vi "Handle Frame.vi"(8 "error in (no error)":errorcluster, 9 "Timeout ms":i32, 10 "Message Frame":T1, 11 "WebSocket Client in":refnum<class "WebSocket Client.lvclass">) -> (0 "error out":errorcluster, 1 "Remaining  Timeout":i32, 3 "WebSocket Client out":refnum<class "WebSocket Client.lvclass">, 4 "Complete":bool)   [LabVIEW 2020, in "HTTP Server.lvlib" / "WebSocket Client.lvclass"]
uses:
  WebSocket Client.lvclass
  WebSocket Client.lvclass/WebSocket Client.ctl
  OpCode.ctl
  Message Frame.ctl
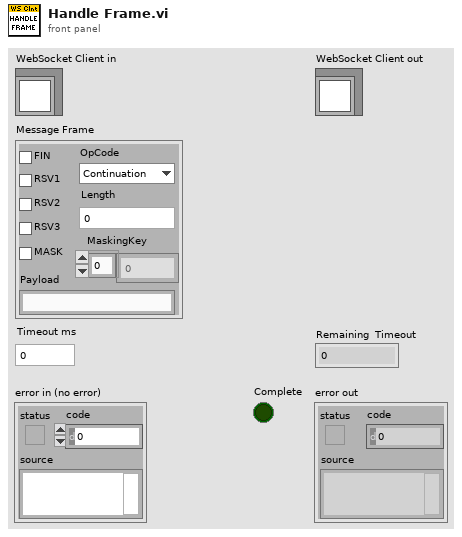
[diagram p1: front panel]
types:
  T1 = typedef "HTTP Server.lvlib/WebSocket Client.lvclass/Message Frame.ctl" = cluster{"FIN":bool, "RSV1":bool, "RSV2":bool, "RSV3":bool, "MASK":bool, "OpCode":T2, "Length":u64, "MaskingKey":u8[], "Payload":string}
  T2 = typedef "HTTP Server.lvlib/WebSocket Client.lvclass/OpCode.ctl" = enum8{"Continuation", "Text", "Binary", "Reserved3", "Reserved4", "Reserved5", "Reserved6", "Reserved7", "Close", "Ping", "Pong", "ReservedB", "ReservedC", "ReservedD", "ReservedE", "ReservedF"}
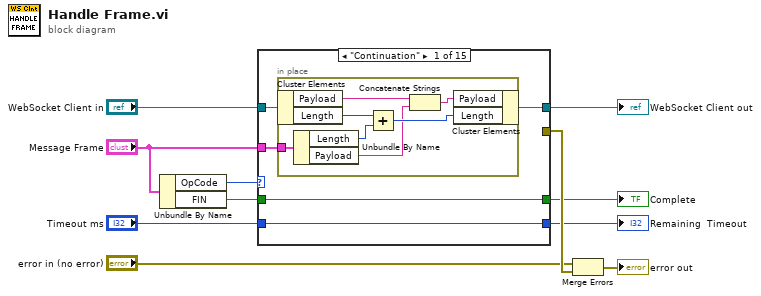
[diagram p0: block diagram]
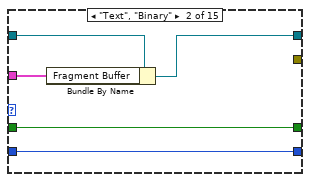
[diagram p2: hidden frame]
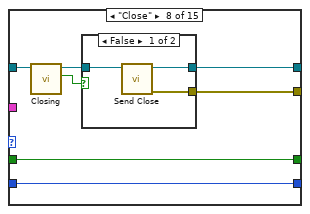
[diagram p8: hidden frame]
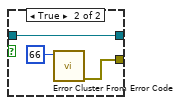
[diagram p9: hidden frame]
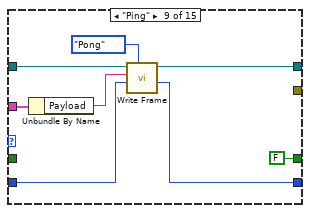
[diagram p10: hidden frame]
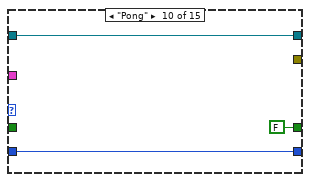
[diagram p11: hidden frame]
diagram:
  n1 = Unbundle By Name("Message Frame") -> ("OpCode"=w9:T2, "FIN"=w8:bool)
  n2 = case shown="\"Continuation\"" w9 {
    tunnel: w8 -> [w12 w27 w30 w33 w36 w39 w42 w49 _ _ w69 w72 w75 w78 w81]
    tunnel: "Timeout ms" -> [w16 w26 w29 w32 w35 w38 w41 w48 w60 w66 w68 w71 w74 w77 w80]
    tunnel: "WebSocket Client in" -> [w15 w28 w31 w34 w37 w40 w43 w50 w64 w67 w70 w73 w76 w79 w82]
    tunnel: [w13 w25 w31 w34 w37 w40 w43 w46 w63 w67 w70 w73 w76 w79 w82] -> w5
    tunnel: [w16 w26 w29 w32 w35 w38 w41 w48 w59 w66 w68 w71 w74 w77 w80] -> w4
    tunnel: "Message Frame" -> [w14 w24 _ _ _ _ _ _ w62 _ _ _ _ _ _]
    tunnel: [w12 w27 w30 w33 w36 w39 w42 w49 FALSE ("FIN") FALSE ("FIN") w69 w72 w75 w78 w81] -> w2
    tunnel: [_ _ _ _ _ _ _ w44 _ _ _ _ _ _ _] -> w11
    frame "Continuation" {
      n3 = in-place {
        in-place-border: w14 -> [w23]
        n4 = in-place-cluster #1(w15) -> ("Payload"=w19:string, "Length"=w22:u64)
        n5 = Unbundle By Name(w23) -> ("Length"=w21:u64, "Payload"=w18:string)
        n6 = Add(x=w22, y=w21) -> (x+y=w20:u64)
        n7 = Concatenate Strings(w19, w18) -> (w17:string)
        n8 = in-place-cluster #1("Payload"=w17, "Length"=w20) -> (w13:refnum<class "WebSocket Client.lvclass">)
      }
    }
    frame "Text", "Binary" {
      n9 = Bundle By Name(cluster=w28, "Fragment Buffer"=w24) -> (w25:refnum<class "WebSocket Client.lvclass">)
    }
    frame "Reserved3" {
    }
    frame "Reserved4" {
    }
    frame "Reserved5" {
    }
    frame "Reserved6" {
    }
    frame "Reserved7" {
    }
    frame "Close" {
      n10 = call "Closing.vi"("WebSocket Client in"=w50) -> ("Closing"=w45:bool, "WebSocket Client out"=w47:refnum<class "WebSocket Client.lvclass">)  [unwired: 8 in, 1 out]
      n11 = case shown="False" w45 {
        tunnel: w47 -> [w53 w56]
        tunnel: [w52 w56] -> w46
        tunnel: [w51 w54] -> w44
        frame False {
          n12 = call "Send Close.vi"("WebSocket Client in"=w53) -> ("error out"=w51:errorcluster, "WebSocket Client out"=w52:refnum<class "WebSocket Client.lvclass">)  [unwired: 9 in]
        }
        frame True {
          n13 = call <vilib>:"Error Cluster From Error Code.vi"("error code (0)"=66) -> ("error out"=w54:errorcluster)  [unwired: 8 in]
        }
      }
    }
    frame "Ping" {
      n14 = Unbundle By Name(w62) -> ("Payload"=w61:string)
      n15 = call "Write Frame.vi"("OpCode"=OpCode."Pong", "Timeout ms"=w60, "Payload"=w61, "WebSocket Client in"=w64) -> ("Remaining  Timeout"=w59:i32, "WebSocket Client out"=w63:refnum<class "WebSocket Client.lvclass">)  [unwired: 5 in, 1 out]
    }
    frame "Pong" {
    }
    frame "ReservedB" {
    }
    frame "ReservedC" {
    }
    frame "ReservedD" {
    }
    frame "ReservedE" {
    }
    frame "ReservedF" {
    }
  }
  "WebSocket Client out" <- w5
  "Complete" <- w2
  "Remaining  Timeout" <- w4
  n16 = Merge Errors("error in (no error)", w11) -> (→"error out":errorcluster)
